vi "Example Callback.vi"() -> ()   [LabVIEW 2013]
uses:
  C:/tf/play/labview/Tinkerforge.dll
  Tinkerforge.dll
panel:
  out "iaqIndexAccuracy":u8
  out "iaqIndex":i32
  out "humidity (%RH)":sgl
  out "airPressure (mbar)":sgl
  in  "stop":bool
  out "temperature (°C)":sgl
  in  "uid":string="abc"
  in  "port":i32=4223
  in  "host":string="localhost"
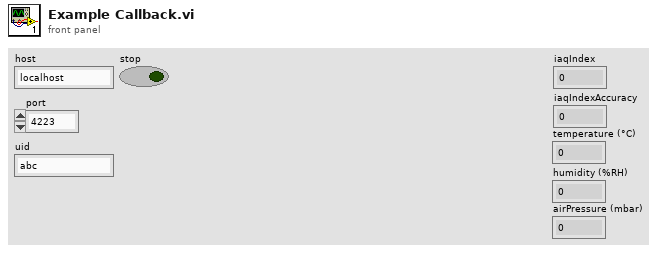
[diagram p1: front panel]
types:
  T1 = cluster{"temperature":i32, "humidity":i32, "airPressure":i32, "iaqIndex":i32, "iaqIndexAccuracy":u8}
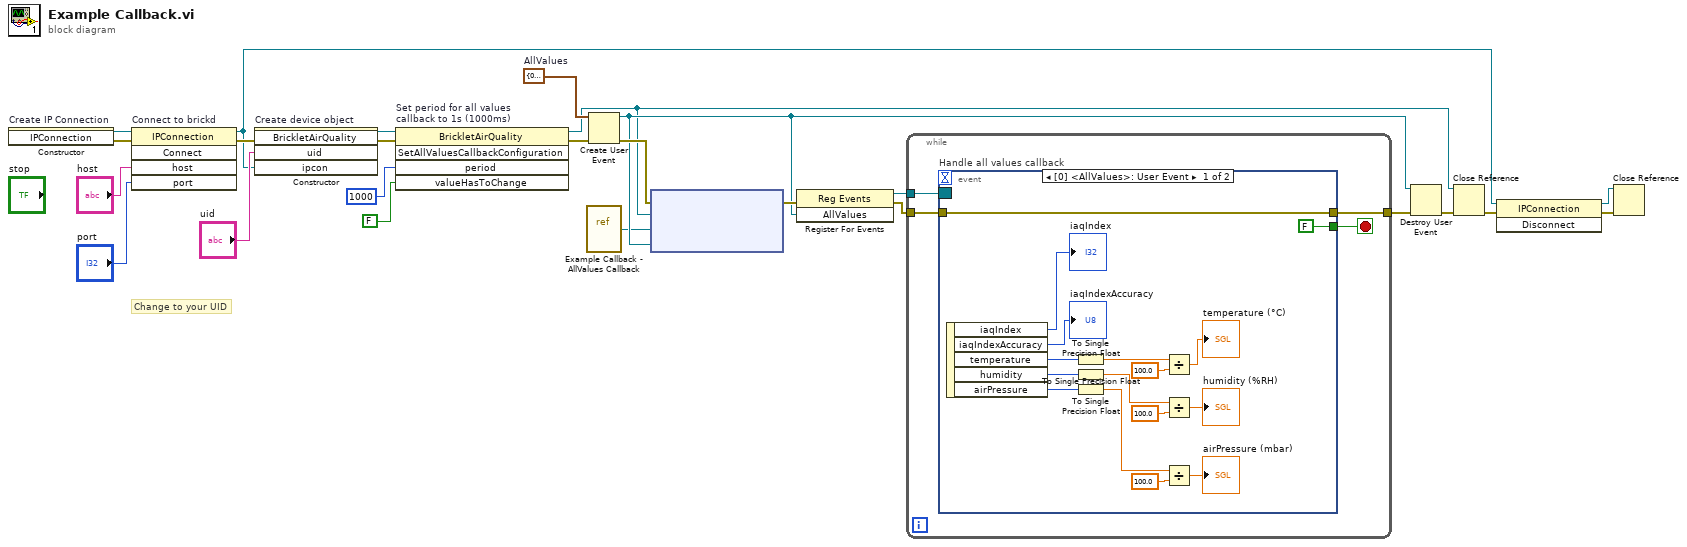
[diagram p0: block diagram]
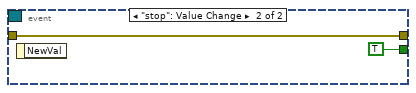
[diagram p2: hidden frame]
diagram:
  w9 = T1 {"temperature"=0, "humidity"=0, "airPressure"=0, "iaqIndex"=0, "iaqIndexAccuracy"=0}  # AllValues
  # "Change to your UID"
  n1 = constructor on="Create IP Connection" class="IPConnection"() -> (reference out=w25:refnum<k24>, error out=w3:errorcluster)  [unwired: 3 in, 1 out]
  n2 = invoke on="Connect to brickd" class="IPConnection" method="Connect"(reference=w25, error in=w3, "host"="host", "port"="port") -> (reference out=w18:refnum<k24>, error out=w21:errorcluster)  [unwired: 1 in, 3 out]
  n3 = constructor on="Create device object" class="BrickletAirQuality"(error in=w21, "uid"="uid", "ipcon"=w18) -> (reference out=w6:refnum<k24>, error out=w8:errorcluster)  [unwired: 2 in, 3 out]
  n4 = invoke on="Set period for all values\ncallback to 1s (1000ms)" class="BrickletAirQuality" method="SetAllValuesCallbackConfiguration"(reference=w6, error in=w8, "period"=i64 1000, "valueHasToChange"=FALSE) -> (reference out=w5:refnum<k24>, error out=w7:errorcluster)  [unwired: 1 in, 3 out]
  n5 = vi-ref "Example Callback - AllValues Callback.vi"() -> ("vi reference"=w1:refnum<vi>)
  n6 = Create User Event(user event datatype=w9, error in=w7) -> (user event=w11:refnum<user-event>, error out=w16:errorcluster)
  n7 = node ("Register Event Callback")(w16, w5, w1, w11) -> (w15:errorcluster)  [unwired: 1 in, 1 out]
  n8 = register-events(error in=w15, w11) -> (reference out=w14:refnum<event-registration>, error out=w12:errorcluster)  [unwired: 1 in]
  n9 = while {
    tunnel: w14 -> [w29]
    tunnel: [w28] -> w13
    tunnel: w12 -> [w27]
    stop <- w26 stop-if-true
    n10 = event "Handle all values callback" shown="[0] <AllValues>: User Event" {
      selector: w29 -> [_ _]
      dyn-events: _ -> [_ _]
      timeout: _ -> [_ _]
      tunnel: [w45 w46] -> w28
      tunnel: w27 -> [w45 w46]
      tunnel: [FALSE TRUE] -> w26
      event User Event {
        n11 = event-data() -> ("iaqIndex"=→"iaqIndex":i32, "iaqIndexAccuracy"=→"iaqIndexAccuracy":u8, "temperature"=w41:i32, "humidity"=w42:i32, "airPressure"=w43:i32)  [unwired: 1 in]
        n12 = To Single Precision Float(number=w41) -> (single precision float=w40:sgl)
        n13 = To Single Precision Float(number=w42) -> (single precision float=w38:sgl)
        n14 = To Single Precision Float(number=w43) -> (single precision float=w36:sgl)
        n15 = Divide(x=w40, y=sgl 100.0) -> (x/y=→"temperature (°C)":sgl)
        n16 = Divide(x=w38, y=sgl 100.0) -> (x/y=→"humidity (%RH)":sgl)
        n17 = Divide(x=w36, y=sgl 100.0) -> (x/y=→"airPressure (mbar)":sgl)
      }
      event "stop": Value Change {
        n18 = event-data() -> ()  [unwired: 1 in, 1 out]
      }
    }
  }
  n19 = Destroy User Event(user event=w11, error in=w13) -> (error out=w10:errorcluster)
  n20 = Close Reference(reference=w5, error in (no error)=w10) -> (error out=w20:errorcluster)
  n21 = invoke class="IPConnection" method="Disconnect"(reference=w18, error in=w20) -> (reference out=w17:refnum<k24>, error out=w19:errorcluster)  [unwired: 1 in, 1 out]
  n22 = Close Reference(reference=w17, error in (no error)=w19) -> ()  [unwired: 1 out]
